vi "SetAnalyzerParameterDirectly.vi"(8 "error in":errorcluster, 10 "Set Parameter List":string[](array[string]), 11 "connection ID in":refnum<k5>) -> (0 "error out":errorcluster, 1 "Error Info":T1, 2 "answer":string, 3 "connection ID out":refnum<k5>, 4 "Log String":string)   [LabVIEW 2020, in "ProdigyRemoteControl.lvlib"]
uses:
  ProdigyRemoteControl.lvlib
  DEFINITIONS/DEF_RcError.ctl
  DEFINITIONS/DEF_RcCmd.ctl
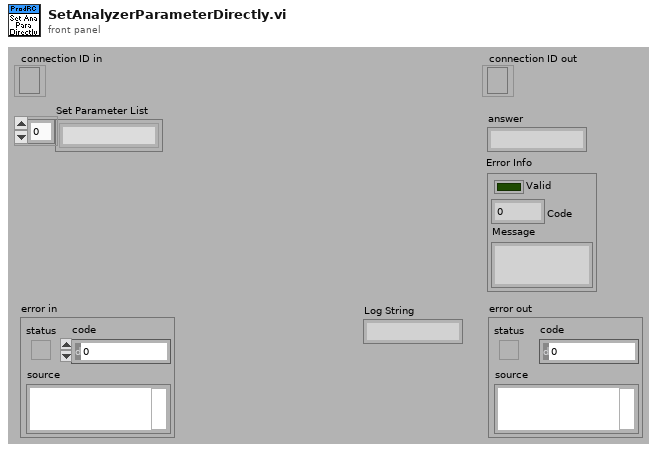
[diagram p1: front panel]
types:
  T1 = typedef "ProdigyRemoteControl.lvlib/DEF_RcError.ctl" = cluster{"Valid":bool, "Code":u16, "Message":string}
  T2 = typedef "ProdigyRemoteControl.lvlib/DEF_RcCmd.ctl" = string
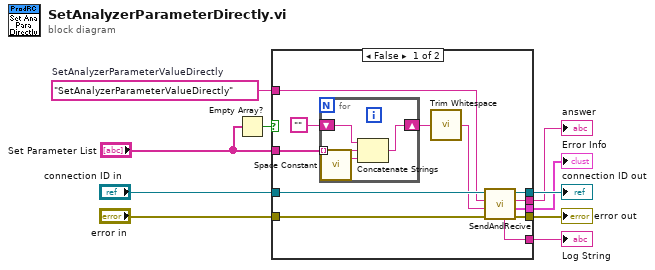
[diagram p0: block diagram]
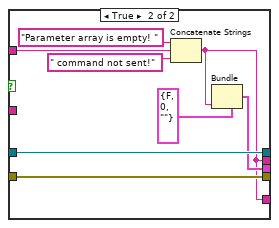
[diagram p2: hidden frame]
diagram:
  w3 = T2 "SetAnalyzerParameterValueDirectly"  # SetAnalyzerParameterValueDirectly
  n1 = Empty Array?(array="Set Parameter List") -> (empty?=w2:bool)
  n2 = case shown="False" w2 {
    tunnel: [w22 w34] -> w10
    tunnel: [w21 w33] -> w9
    tunnel: "error in" -> [w20 w33]
    tunnel: "connection ID in" -> [w19 w34]
    tunnel: [w18 w27] -> w6
    tunnel: [w17 w28] -> w5
    tunnel: [w16 w27] -> w4
    tunnel: "Set Parameter List" -> [w15 _]
    tunnel: w3 -> [w11 w31]
    frame False {
      n3 = for {
        tunnel: w15 -> [w26] mode=indexing
        shift-right: [w23] -> w13
        shift-left: "" -> [w24]
        n4 = call <vilib>:"Space Constant.vi"() -> ("String"=w25:string)
        n5 = Concatenate Strings(w24, w26, w25) -> (w23:string)
      }
      n6 = call <vilib>:"Trim Whitespace.vi"("string"=w13) -> ("trimmed string"=w12:string)  [unwired: 1 in]
      n7 = call "SendAndRecive.vi"("error in"=w20, "Parameters"=w12, "Command"=w11, "connection ID in"=w19) -> ("error out"=w21:errorcluster, "Error Info"=w17:T1, "Answer"=w18:string, "connection ID out"=w22:refnum<k5>, "Log String"=w16:string)  [unwired: 3 in]
    }
    frame True {
      n8 = Concatenate Strings("Parameter array is empty! " ("string"), w31, " command not sent!" ("string")) -> (w27:string)
      n9 = Bundle(cluster=T1 {"Valid"=FALSE, "Code"=0, "Message"=""} ("Error Info"), "Message"=w27) -> (w28:T1)  [unwired: 2 in]
    }
  }
  "connection ID out" <- w10
  "error out" <- w9
  "answer" <- w6
  "Error Info" <- w5
  "Log String" <- w4
